vi "PosStrikerFollowAttacker.vi"(4 "Pos Attacker":dbl[](array[numeric]), 6 "atacando ao contrário?":bool=TRUE, 7 "AI Parameters":T4={"GotoKick"={"Dist do cone a frente"=150.0, "attacker farback"=1500.0, "Perto"=300.0, "min dist to kick"=150.0, "kick eps"=0.0, "Time to transition"=0.05}, "Attacker"={"CC chute"=0.09, "CC passe"=0.045, "Kick Force"=100.0, "D ball-robot Kick"=200.0, "D ball-robot Pass"=0.3}, "Defender"={"D max"=1700.0, "Vel p/ robô av"=1000.0, "Kick Force"=100.0, "D atk-def"=0.0, "D farback"=0.0}, "Timeout"={"Field/v in x"=6.0, "Dist Robots"=300, "Dist up in y"=300}, "Pose Striker"={"dist"=200.0, "Numeric"=-4.0, "dist 2"=200.0}, "Dist Stop"=300.0, "Distance when ball out"=200, "D central gap "=150.0, "T pass"=0.0, "Force ++"=0.0, "range kick"=0.0, "Chute alto"=TRUE, "Marcador novo"=TRUE} {"D central gap" format="%#_13g"; "Dist Stop" format="%#_13g"; "Pose Striker"."Numeric" format="%#_13g"; "Defender"."Kick Force" format="%#_13g"; "Defender"."Vel p/ robô av" format="%#_13g"; "Attacker"."D ball-robot Kick" format="%#_13g"; "Attacker"."Kick Force" format="%#_13g"; "Attacker"."CC passe" format="%#_13g"; "Attacker"."CC chute" format="%#_13g"; "GotoKick"."kick eps" format="%#_13g"; "GotoKick"."min dist to kick" format="%#_13g"; "GotoKick"."Perto" format="%#_13g"; "GotoKick"."attacker farback" format="%#_13g"; "GotoKick"."Dist do cone a frente" format="%#_13g"}, 8 "IA Input":T5={"our_robots"=[], "enemy_robots"=[], "balls"=[], "geometry"={"line_width"=0, "field_length"=0, "field_width"=0, "boundary_width"=0, "referee_width"=0, "goal_width"=0, "goal_depth"=0, "goal_wall_width"=0, "center_circle_radius"=0, "defense_radius"=0, "defense_stretch"=0, "free_kick_from_defense_dist"=0, "penalty_spot_from_field_line_dist"=0, "penalty_line_from_spot_dist"=0}, "IA Judge"={"stage"="", "command"="", "our_goalie_id"=0.0, "enemy_goalie_id"=0.0, "command enum"=enum."Halt", "Time"=enum."Azul"}, "Received Timestamp"=timestamp(0 s since 1904-01-01), "Events"={"Touch"=FALSE, "Ball out"=FALSE, "id touch"=0.0, "Ball out of \nVision"=FALSE, "Ball inside \nGoalie area"=FALSE, "Robot not responding"=FALSE, "Robots responding status"=[1.0, 1.0, 1.0, 1.0, 1.0, 1.0], "Enemy Ball \nPossession"=FALSE, "Pass State"=FALSE, "id end of pass"=0.0, "Kick"=FALSE, "Id ini Possession"=0.0, "Ball Possesion"=FALSE, "Id Possesion"=0.0}}, 9 "balls":T6[](array[typedef])=[{"x"=-2165.869384765625, "y"=510.4085693359375, "timestamp"=timestamp(2082758857.4639893 s since 1904-01-01), "Vel_x"=0.0, "Vel_y"=0.0, "Pos Bola Est"=[]}], 10 "Field Size in":T7={"line_width"=10, "field_length"=6000, "field_width"=4000, "boundary_width"=250, "referee_width"=425, "goal_width"=700, "goal_depth"=180, "goal_wall_width"=20, "center_circle_radius"=500, "defense_radius"=500, "defense_stretch"=350, "free_kick_from_defense_dist"=700, "penalty_spot_from_field_line_dist"=450, "penalty_line_from_spot_dist"=350}, 11 "Robot":T1={"id"=0, "function"=enum."Attacker", "x"=0.0, "y"=0.0, "orientation"=0.0, "v_tangent"=0.0, "v_normal"=0.0, "v_ang"=0.0, "kick_x"=0.0, "kick_z"=0.0, "dribble"=FALSE, "Timestamp"=timestamp(0 s since 1904-01-01), "dest_x"=0.0, "dest_y"=0.0, "dest_orientation"=0.0, "estimatives"={"est_v_tangent"=0.0, "est_v_normal"=0.0, "est_vx"=0.0, "est_vy"=0.0, "Pos Robot Est"=[]}, "dest_x_kick"=0.0, "dest_y_kick"=0.0, "Gap Coord"=[], "States"=enum."GoToTangent"}) -> (2 "Robot 2":T1={"id"=0, "function"=enum."Attacker", "x"=0.0, "y"=0.0, "orientation"=0.0, "v_tangent"=0.0, "v_normal"=0.0, "v_ang"=0.0, "kick_x"=0.0, "kick_z"=0.0, "dribble"=FALSE, "Timestamp"=timestamp(0 s since 1904-01-01), "dest_x"=0.0, "dest_y"=0.0, "dest_orientation"=0.0, "estimatives"={"est_v_tangent"=0.0, "est_v_normal"=0.0, "est_vx"=0.0, "est_vy"=0.0, "Pos Robot Est"=[]}, "dest_x_kick"=0.0, "dest_y_kick"=0.0, "Gap Coord"=[], "States"=enum."GoToTangent"})   [LabVIEW 2016]
uses:
  Core/Field Size.ctl
  Core/AI Ball.ctl
  Core/AI Input.ctl
  Core/AI Robot.ctl
  Functions Enum.ctl
  AttackerStates.ctl
  Core/AI Judge.ctl
  Command Enum.ctl
  Util/Events/Events.ctl
  AI Parameters.ctl
panel:
  out "sentido":dbl
  out "Yattacker":dbl
  out "Xattacker":dbl
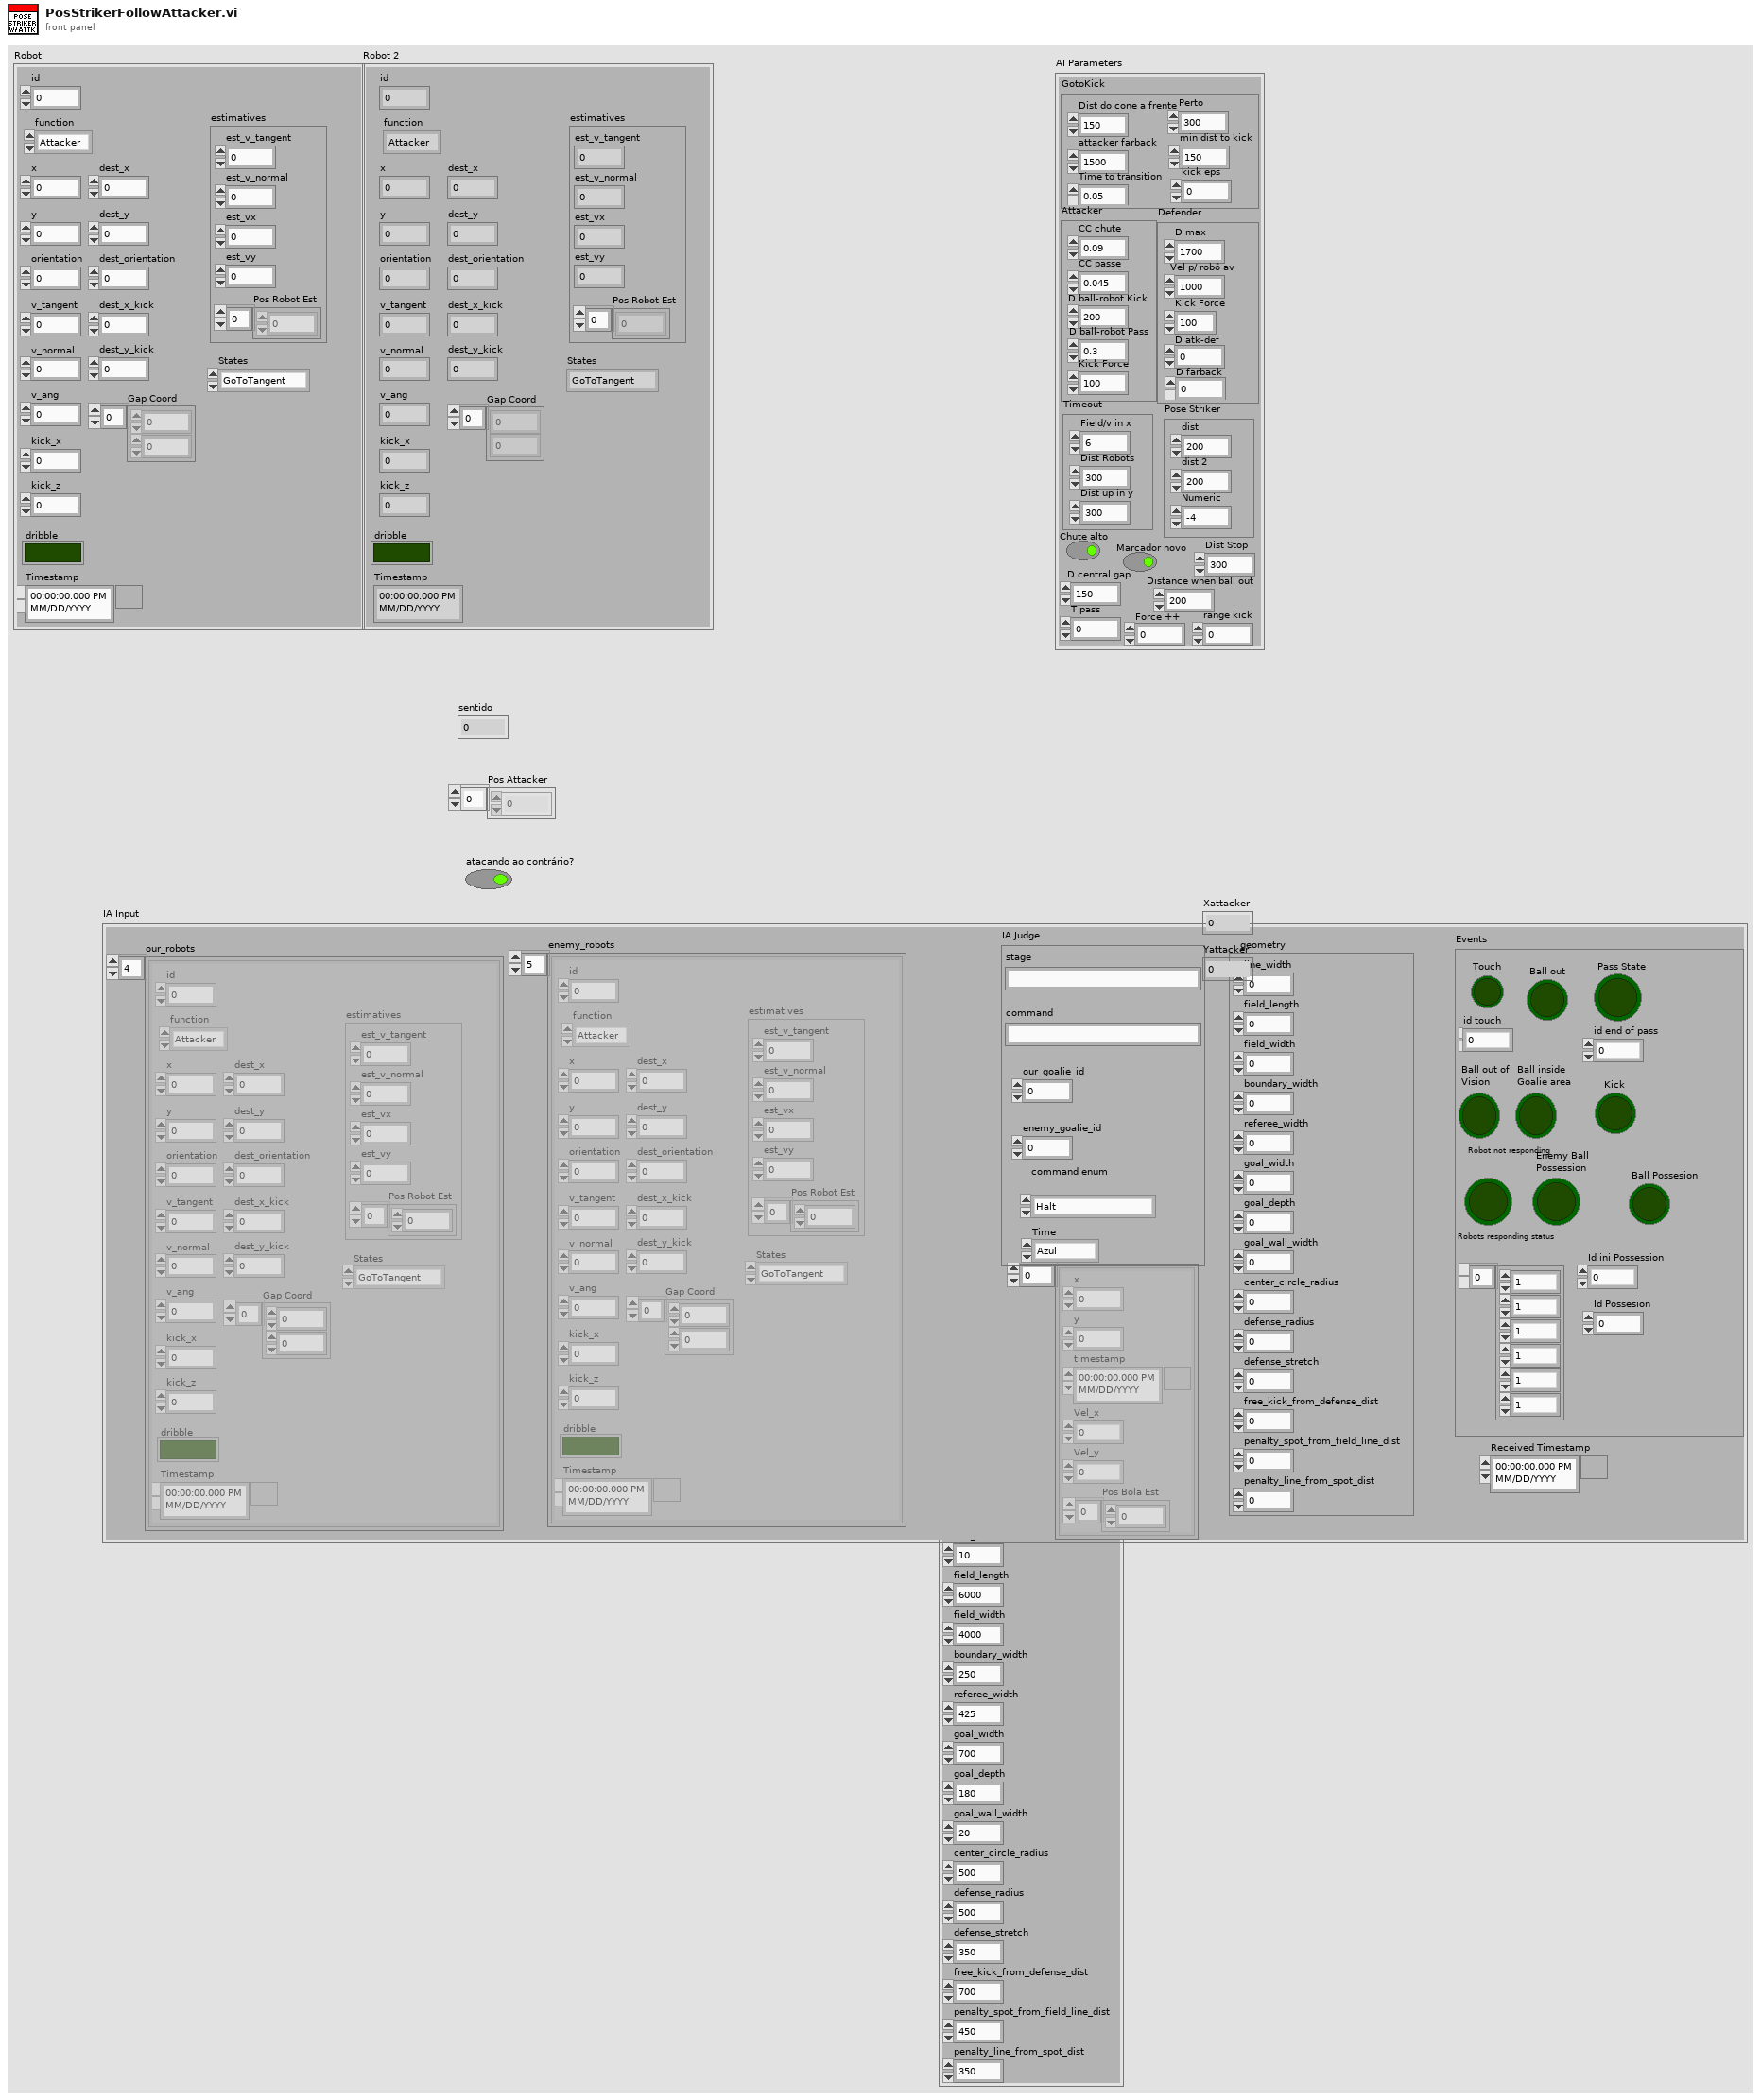
[diagram p1: front panel]
types:
  T1 = typedef "AI Robot.ctl" = cluster{"id":u32, "function":T2, "x":dbl, "y":dbl, "orientation":dbl, "v_tangent":dbl, "v_normal":dbl, "v_ang":dbl, "kick_x":dbl, "kick_z":dbl, "dribble":bool, "Timestamp":timestamp, "dest_x":dbl, "dest_y":dbl, "dest_orientation":dbl, "estimatives":cluster{"est_v_tangent":dbl, "est_v_normal":dbl, "est_vx":dbl, "est_vy":dbl, "Pos Robot Est":dbl[]}, "dest_x_kick":dbl, "dest_y_kick":dbl, "Gap Coord":dbl[], "States":T3}
  T2 = typedef "Functions Enum.ctl" = enum16{"Attacker", "Goalie", "Defender", "Striker", "Goto 0", "Dummy", "Kicker", "ZigZag"}
  T3 = typedef "AttackerStates.ctl" = enum16{"Pass", "GoToTangent", "BallGetting", "GoToKick", ""}
  T4 = typedef "AI Parameters.ctl" = cluster{"GotoKick":cluster{"Dist do cone a frente":dbl, "attacker farback":dbl, "Perto":dbl, "min dist to kick":dbl, "kick eps":dbl, "Time to transition":dbl}, "Attacker":cluster{"CC chute":dbl, "CC passe":dbl, "Kick Force":dbl, "D ball-robot Kick":dbl, "D ball-robot Pass":dbl}, "Defender":cluster{"D max":dbl, "Vel p/ robô av":dbl, "Kick Force":dbl, "D atk-def":dbl, "D farback":dbl}, "Timeout":cluster{"Field/v in x":dbl, "Dist Robots":u32, "Dist up in y":u32}, "Pose Striker":cluster{"dist":dbl, "Numeric":dbl, "dist 2":dbl}, "Dist Stop":dbl, "Distance when ball out":i32, "D central gap ":dbl, "T pass":dbl, "Force ++":dbl, "range kick":dbl, "Chute alto":bool, "Marcador novo":bool}
  T5 = typedef "AI Input.ctl" = cluster{"our_robots":T1[], "enemy_robots":T1[], "balls":T6[], "geometry":T7, "IA Judge":T8, "Received Timestamp":timestamp, "Events":T10}
  T6 = typedef "AI Ball.ctl" = cluster{"x":dbl, "y":dbl, "timestamp":timestamp, "Vel_x":dbl, "Vel_y":dbl, "Pos Bola Est":dbl[]}
  T7 = typedef "Field Size.ctl" = cluster{"line_width":u32, "field_length":u32, "field_width":u32, "boundary_width":u32, "referee_width":u32, "goal_width":u32, "goal_depth":u32, "goal_wall_width":u32, "center_circle_radius":u32, "defense_radius":u32, "defense_stretch":u32, "free_kick_from_defense_dist":u32, "penalty_spot_from_field_line_dist":u32, "penalty_line_from_spot_dist":u32}
  T8 = typedef "AI Judge.ctl" = cluster{"stage":string, "command":string, "our_goalie_id":dbl, "enemy_goalie_id":dbl, "command enum":T9, "Time":enum16{"Azul", "Amarelo"}}
  T9 = typedef "Command Enum.ctl" = enum16{"Halt", "Stop", "Force Start", "PKA Normal Start", "Prepare Kickoff Ally", "PKE Normal Start", "Prepare Kickoff Enemy", "Prepare Penalty Ally", "PPA Normal Start", "Prepare Penalty Enemy", "PPE Normal Start", "Direct Free Enemy", "Direct Free Ally", "Indirect Free Enemy", "Indirect Free Ally", "Timeout Enemy", "Timeout Ally", "Goal Enemy", "Goal Ally", "Ball Placement Enemy", "Ball Placement Ally", "Normal Half Time", "Extra Time Break", "Extra Half Time", "None", "Post Game"}
  T10 = typedef "Events.ctl" = cluster{"Touch":bool, "Ball out":bool, "id touch":dbl, "Ball out of \nVision":bool, "Ball inside \nGoalie area":bool, "Robot not responding":bool, "Robots responding status":dbl[], "Enemy Ball \nPossession":bool, "Pass State":bool, "id end of pass":dbl, "Kick":bool, "Id ini Possession":dbl, "Ball Possesion":bool, "Id Possesion":dbl}
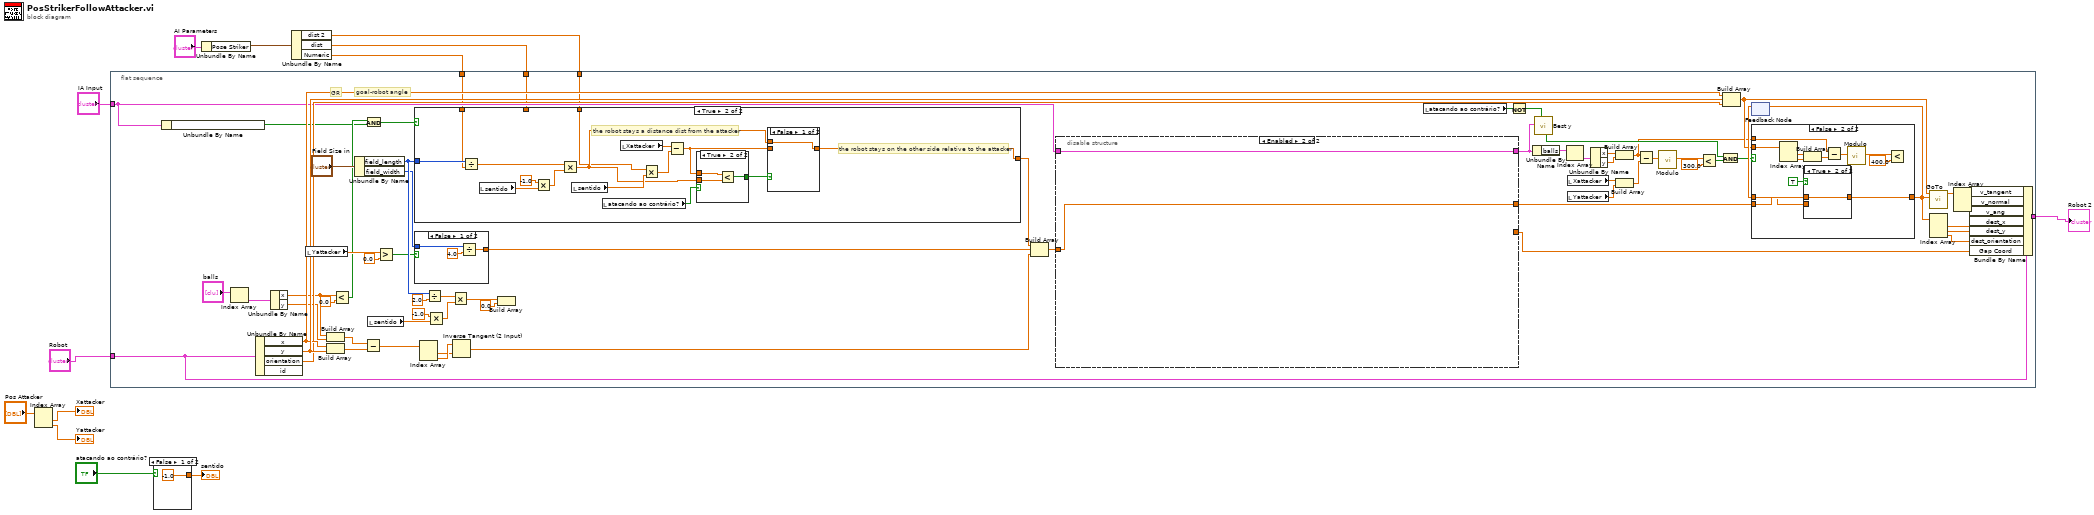
[diagram p0: block diagram]
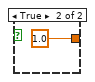
[diagram p2: hidden frame]
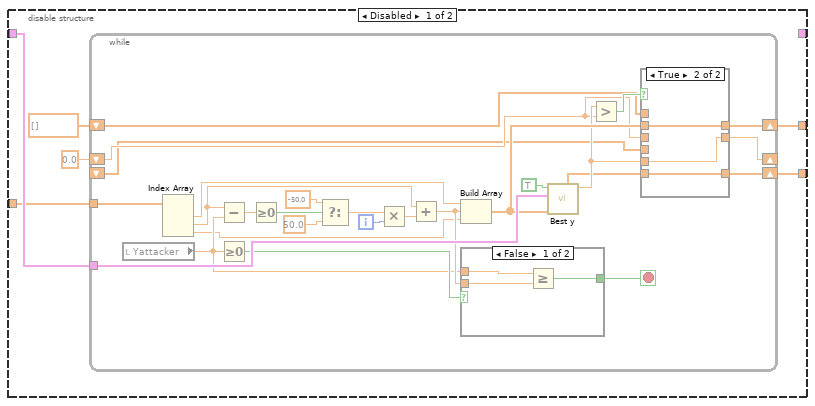
[diagram p5: hidden frame]
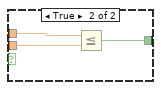
[diagram p6: hidden frame]
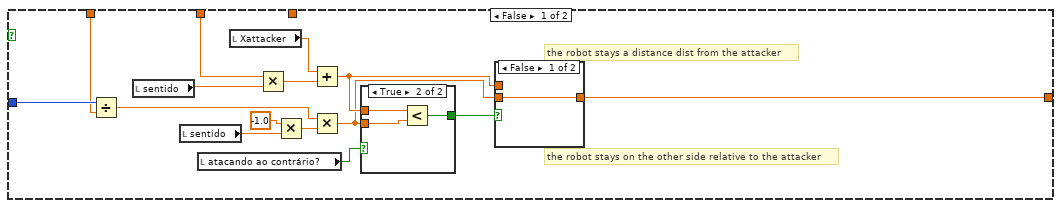
[diagram p8: hidden frame]
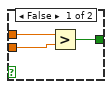
[diagram p9: hidden frame]
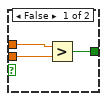
[diagram p11: hidden frame]
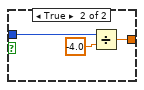
[diagram p13: hidden frame]
diagram:
  n1 = Index Array(array="Pos Attacker") -> (element #1=→"Xattacker":dbl, element #2=→"Yattacker":dbl)  [unwired: 2 in]
  n2 = flat-sequence {
    tunnel: [w61] -> w1
    tunnel: "Robot" -> [w59]
    tunnel: "IA Input" -> [w19]
    tunnel: w7 -> [w16]
    tunnel: w6 -> [w15]
    tunnel: w5 -> [w14]
    frame #0 {
      # "GR"
      # "goal-robot angle"
      n3 = Unbundle By Name(w19) -> ("Events.Ball inside \nGoalie area"=w45:bool)
      n4 = Index Array(array="balls") -> (element=w49:T6)  [unwired: 1 in]
      n5 = Unbundle By Name(w59) -> ("x"=w75:dbl, "y"=w76:dbl, "orientation"=w62:dbl)  [unwired: 1 out]
      n6 = Unbundle By Name(w49) -> ("x"=w43:dbl, "y"=w42:dbl)
      n7 = local read "Yattacker"() -> (w60:dbl)
      n8 = Build Array(w43, w42) -> (w41:dbl[])
      n9 = Build Array(w75, w76) -> (w77:dbl[])
      n10 = Less?(x=w43, y=0.0) -> (x < y?=w46:bool)
      n11 = Unbundle By Name("Field Size in") -> ("field_length"=w79:u32, "field_width"=w66:u32)
      n12 = Subtract(x=w41, y=w77) -> (x-y=w74:dbl[])
      n13 = And(x=w46, y=w45) -> (x .and. y?=w47:bool)
      n14 = local read "sentido"() -> (w57:dbl)
      n15 = Greater?(x=w60, y=0.0) -> (0:w63:bool)
      n16 = case shown="True" w47 {
        tunnel: w79 -> [w158 w181]
        tunnel: [w157 w180] -> w68
        tunnel: w16 -> [w145 _]
        tunnel: w15 -> [w144 w168]
        tunnel: w14 -> [_ w167]
        frame False {
          # "the robot stays on the other side relative to the attacker"
          # "the robot stays a distance dist from the attacker"
          n17 = Divide(x=w158, y=w144) -> (x/y=w156:dbl)
          n18 = local read "sentido"() -> (w150:dbl)
          n19 = local read "sentido"() -> (w153:dbl)
          n20 = local read "atacando ao contrário?"() -> (w149:bool)
          n21 = local read "Xattacker"() -> (w155:dbl)
          n22 = Multiply(x=w145, y=w150) -> (x*y=w154:dbl)
          n23 = Multiply(x=-1.0, y=w153) -> (x*y=w152:dbl)
          n24 = Add(x=w155, y=w154) -> (x+y=w148:dbl)
          n25 = Multiply(x=w156, y=w152) -> (x*y=w147:dbl)
          n26 = case shown="True" w149 {
            tunnel: w148 -> [w161 w163]
            tunnel: w147 -> [w160 w164]
            tunnel: [w159 w162] -> w146
            frame False {
              n27 = Greater?(x=w161, y=w160) -> (0:w159:bool)
            }
            frame True {
              n28 = Less?(x=w163, y=w164) -> (x < y?=w162:bool)
            }
          }
          n29 = case shown="False" w146 {
            tunnel: [w165 w166] -> w157
            tunnel: w148 -> [_ w166]
            tunnel: w147 -> [w165 _]
            frame False {
            }
            frame True {
            }
          }
        }
        frame True {
          # "the robot stays on the other side relative to the attacker"
          # "the robot stays a distance dist from the attacker"
          n30 = Divide(x=w181, y=w168) -> (x/y=w179:dbl)
          n31 = local read "sentido"() -> (w176:dbl)
          n32 = Multiply(x=-1.0, y=w176) -> (x*y=w175:dbl)
          n33 = Multiply(x=w179, y=w175) -> (x*y=w170:dbl)
          n34 = local read "sentido"() -> (w173:dbl)
          n35 = local read "atacando ao contrário?"() -> (w172:bool)
          n36 = local read "Xattacker"() -> (w178:dbl)
          n37 = Multiply(x=w167, y=w173) -> (x*y=w177:dbl)
          n38 = Subtract(x=w178, y=w177) -> (x-y=w171:dbl)
          n39 = case shown="True" w172 {
            tunnel: w171 -> [w184 w186]
            tunnel: w170 -> [w183 w187]
            tunnel: [w182 w185] -> w169
            frame False {
              n40 = Greater?(x=w184, y=w183) -> (0:w182:bool)
            }
            frame True {
              n41 = Less?(x=w186, y=w187) -> (x < y?=w185:bool)
            }
          }
          n42 = case shown="False" w169 {
            tunnel: [w188 w189] -> w180
            tunnel: w171 -> [_ w189]
            tunnel: w170 -> [w188 _]
            frame False {
            }
            frame True {
            }
          }
        }
      }
      n43 = case shown="False" w63 {
        tunnel: [w191 w194] -> w67
        tunnel: w66 -> [w190 w193]
        frame False {
          n44 = Divide(x=w190, y=4.0) -> (x/y=w191:dbl)
        }
        frame True {
          n45 = Divide(x=w193, y=-4.0) -> (x/y=w194:dbl)
        }
      }
      n46 = Index Array(array=w74) -> (element #1=w72:dbl, element #2=w73:dbl)  [unwired: 2 in]
      n47 = Divide(x=w79, y=2.0) -> (x/y=w55:dbl)
      n48 = Multiply(x=-1.0, y=w57) -> (x*y=w56:dbl)
      n49 = Multiply(x=w55, y=w56) -> (x*y=w54:dbl)
      n50 = Inverse Tangent (2 Input)(1:w72, 2:w73) -> (0:w81:dbl)
      n51 = Build Array(w54, 0.0 ("element")) -> ()  [unwired: 1 out]
      n52 = Build Array(w68, w67, w81) -> (w44:dbl[])
      n53 = disable-structure shown="Enabled" {
        disable-tunnel: w19 -> [w102 w142]
        disable-tunnel: w44 -> [w101 w143]
        disable-tunnel: [w100 w143] -> w40
        disable-tunnel: [w97 _] -> w18
        disable-tunnel: [_ w142] -> w35
        frame Disabled {
          n54 = while {
            tunnel: w102 -> [w124]
            shift-right: [w122] -> w100
            shift-left: dbl[] [] -> [w117]
            shift-right: [w120] -> _
            shift-left: 0.0 ("Gap kick") -> [w118]
            tunnel: w101 -> [w107]
            shift-right: [w106] -> w97
            shift-left: _ -> [w105]
            i -> [w127]
            stop <- w126 stop-if-true
            n55 = local read "Yattacker"() -> (w108:dbl)
            n56 = Index Array(array=w107) -> (element #1=w128:dbl, element #2=w116:dbl, element #3=w103:dbl)  [unwired: 3 in]
            n57 = Subtract(x=w116, y=w108) -> (x-y=w115:dbl)
            n58 = Greater Or Equal To 0?(x=w108) -> (x >= 0?=w109:bool)
            n59 = Greater Or Equal To 0?(x=w115) -> (x >= 0?=w114:bool)
            n60 = Select(t=-50.0, s=w114, f=50.0) -> (s? t:f=w111:dbl)
            n61 = Multiply(x=w111, y=w127) -> (x*y=w125:dbl)
            n62 = Add(x=w116, y=w125) -> (x+y=w110:dbl)
            n63 = Build Array(w128, w110, w103) -> (w123:dbl[])
            n64 = case shown="False" w109 {
              tunnel: [w132 w135] -> w126
              tunnel: w108 -> [w131 w134]
              tunnel: w110 -> [w130 w133]
              frame False {
                n65 = Greater Or Equal?(x=w131, y=w130) -> (x >= y?=w132:bool)
              }
              frame True {
                n66 = Less Or Equal?(x=w134, y=w133) -> (x <= y?=w135:bool)
              }
            }
            n67 = call "Best y.vi"("Ball false"=w123, "IA State"=w124, "Best y para varredura?"=TRUE) -> ("Gap kick"=w119:dbl, "Gap Coord"=w104:dbl[])  [unwired: 5 in, 2 out]
            n68 = Greater?(x=w119, y=w118) -> (0:w121:bool)
            n69 = case shown="True" w121 {
              tunnel: w123 -> [_ w141]
              tunnel: [w137 w141] -> w122
              tunnel: [w138 w140] -> w120
              tunnel: w119 -> [_ w140]
              tunnel: w118 -> [w138 _]
              tunnel: w117 -> [w137 _]
              tunnel: [w136 w139] -> w106
              tunnel: w105 -> [w136 _]
              tunnel: w104 -> [_ w139]
              frame False {
              }
              frame True {
              }
            }
          }
        }
        frame Enabled {
        }
      }
      n70 = local read "atacando ao contrário?"() -> (w36:bool)
      n71 = Not(x=w36) -> (.not. x?=w37:bool)
      n72 = Unbundle By Name(w35) -> ("balls"=w34:T6[])
      n73 = call "Best y.vi"("inimigos"=w37, "IA State"=w35) -> ("Eclipse"=w26:bool)  [unwired: 6 in, 3 out]
      n74 = Index Array(array=w34) -> (element=w33:T6)  [unwired: 1 in]
      n75 = local read "Xattacker"() -> (w30:dbl)
      n76 = local read "Yattacker"() -> (w29:dbl)
      n77 = Unbundle By Name(w33) -> ("x"=w32:dbl, "y"=w31:dbl)
      n78 = Build Array(w32, w31) -> (w20:dbl[])
      n79 = Build Array(w30, w29) -> (w28:dbl[])
      n80 = Subtract(x=w20, y=w28) -> (x-y=w27:dbl[])
      n81 = call "Modulo.vi"("2D vector"=w27) -> ("Modulo"=w23:dbl)  [unwired: 10 in]
      n82 = Less?(x=w23, y=300.0 ("x")) -> (x < y?=w24:bool)
      n83 = And(x=w26, y=w24) -> (x .and. y?=w25:bool)
      n84 = Build Array(w75, w76, w62) -> (w21:dbl[])
      n85 = feedback #1() -> (w38:dbl[])  [unwired: 1 in]
      n86 = case shown="False" w25 {
        tunnel: w40 -> [_ w85]
        tunnel: [w82 w86] -> w39
        tunnel: w38 -> [w82 w84]
        tunnel: w21 -> [_ w94]
        tunnel: w20 -> [_ w91]
        frame True {
        }
        frame False {
          n87 = Index Array(array=w94) -> (element #1=w93:dbl, element #2=w92:dbl)  [unwired: 2 in]
          n88 = Build Array(w93, w92) -> (w90:dbl[])
          n89 = case shown="True" TRUE {
            tunnel: [w95 w96] -> w86
            tunnel: w85 -> [_ w96]
            tunnel: w84 -> [w95 _]
            frame False {
            }
            frame True {
            }
          }
          n90 = Subtract(x=w91, y=w90) -> (x-y=w89:dbl[])
          n91 = call "Modulo.vi"("2D vector"=w89) -> ("Modulo"=w88:dbl)  [unwired: 10 in]
          n92 = Less?(x=w88, y=400.0) -> ()  [unwired: 1 out]
        }
      }
      n93 = feedback-in #1(w39) -> ()
      n94 = call "GoTo.vi"("Target"=w39, "Position"=w21) -> ("Output\nVelocity"=w53:dbl[])  [unwired: 8 in, 1 out]
      n95 = Index Array(array=w39) -> (element #1=w52:dbl, element #2=w51:dbl, element #3=w17:dbl)  [unwired: 3 in]
      n96 = Index Array(array=w53) -> (element #1=w69:dbl, element #2=w71:dbl, element #3=w70:dbl)  [unwired: 3 in]
      n97 = Bundle By Name(cluster=w59, "v_tangent"=w69, "v_normal"=w71, "v_ang"=w70, "dest_x"=w52, "dest_y"=w51, "dest_orientation"=w17, "Gap Coord"=w18) -> (w61:T1)
    }
  }
  n98 = case shown="False" "atacando ao contrário?" {
    tunnel: [-1.0 1.0] -> w12
    frame False {
    }
    frame True {
    }
  }
  "sentido" <- w12
  n99 = Unbundle By Name("AI Parameters") -> ("Pose Striker"=w3:cluster{"dist":dbl, "Numeric":dbl, "dist 2":dbl})
  n100 = Unbundle By Name(w3) -> ("dist 2"=w5:dbl, "dist"=w7:dbl, "Numeric"=w6:dbl)
  "Robot 2" <- w1
